vi "SQL_在指定表中指定字段插入多条数据.vi"(8 "error in (no error)":errorcluster caption="错误输入（无错误）", 9 "字段值(字符)":string[][](array[string]), 10 "字段名(字符)":string[](array[string]), 11 "表名":string="d7") -> (0 "error out":errorcluster caption="错误输出", 3 "SQL_在指定表中指定字段插入数据":string)   [LabVIEW 2014]
doc: "该模板用于创建子VI。"
uses:
  <vilib>/addons/database/NI_Database_API.lvlib
  <vilib>/addons/database/Connection.llb/DB Tools Open Connec (String).vi
  <vilib>/addons/database/Connection.llb/Conn Execute.vi
  <vilib>/addons/database/Recordset.llb/Rec Destroy - Connection.vi
panel:
  out "error out 2":errorcluster
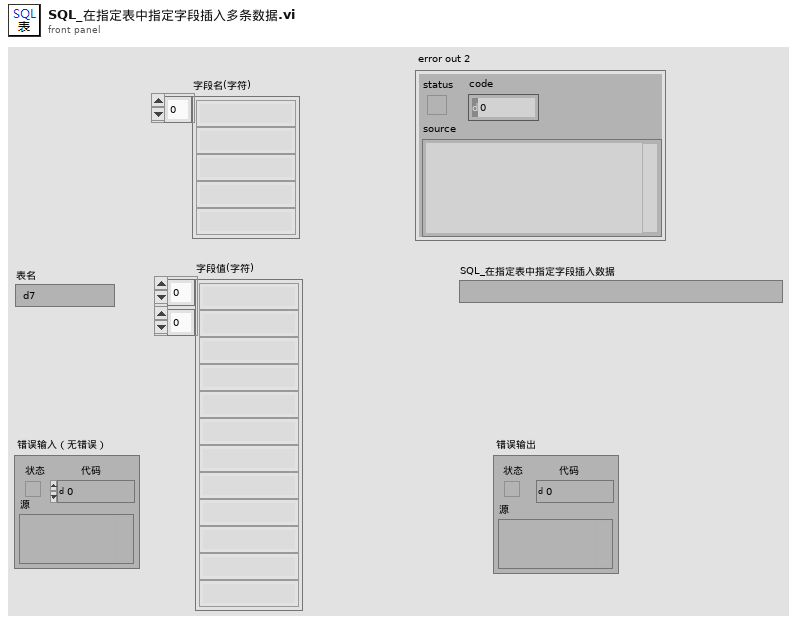
[diagram p1: front panel]
types:
  T1 = typedef "NI_Database_API.lvlib/Conn ObjectReference.ctl" = refnum<k1>
  T2 = typedef "NI_Database_API.lvlib/Rec ObjectReference.ctl" = refnum<k1>
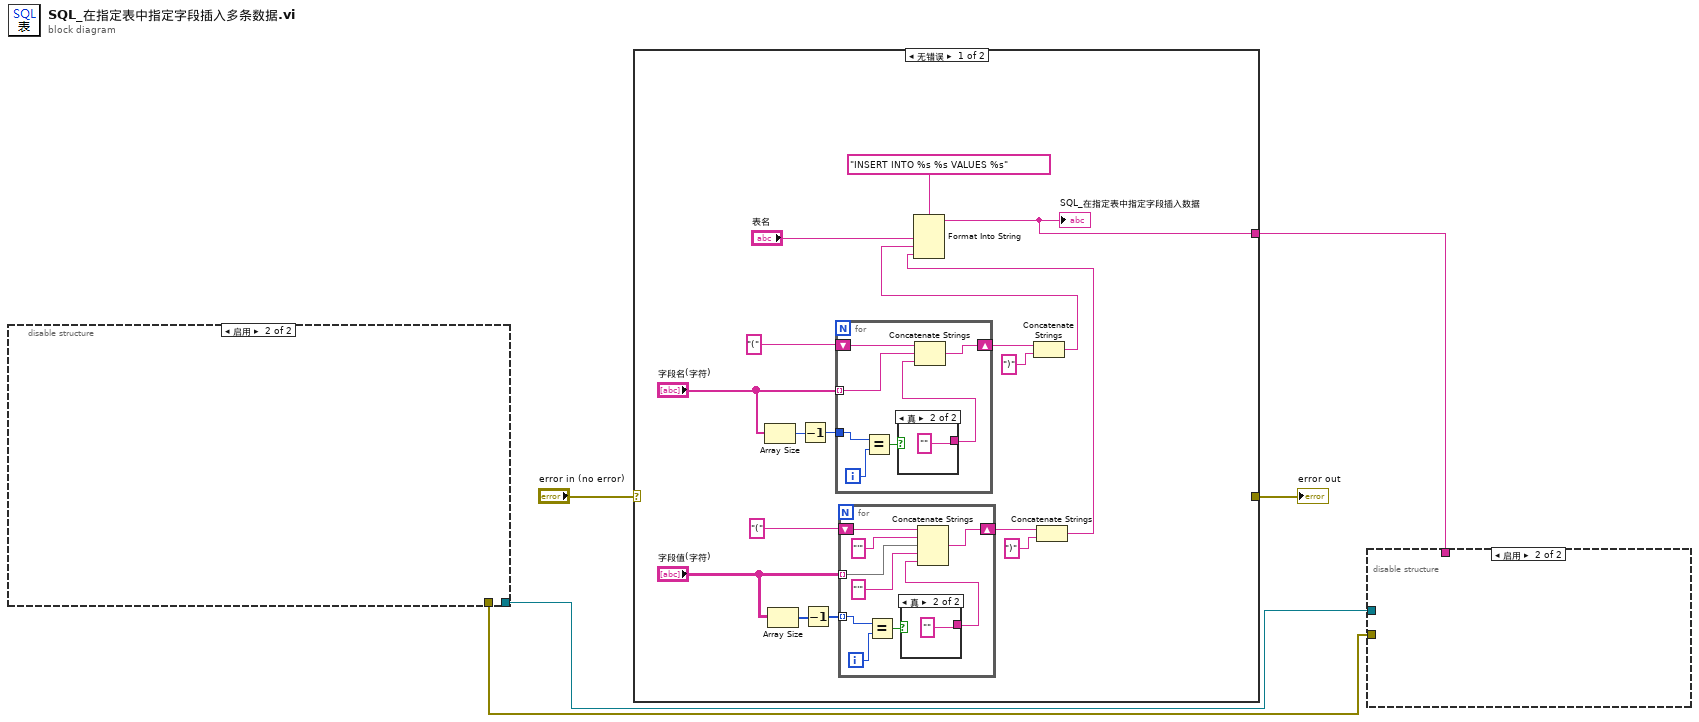
[diagram p0: block diagram]
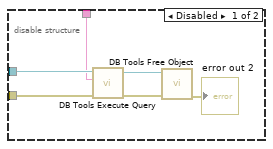
[diagram p2: hidden frame]
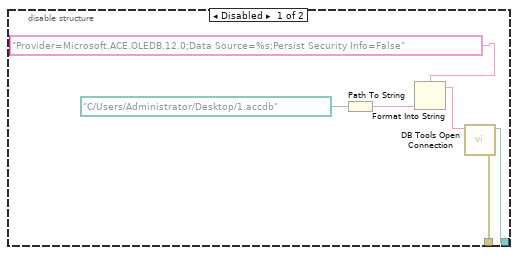
[diagram p3: hidden frame]
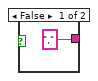
[diagram p4: hidden frame]
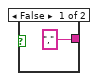
[diagram p5: hidden frame]
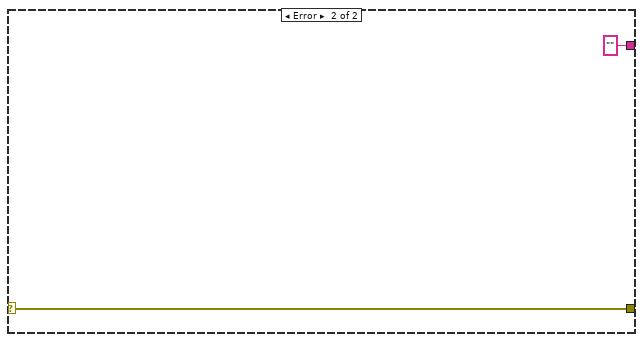
[diagram p6: hidden frame]
diagram:
  n1 = disable-structure shown="启用" {
    disable-tunnel: [w8 _] -> w3
    disable-tunnel: [w6 _] -> w2
    frame Disabled {
      n2 = Path To String(path=path "C:/Users/Administrator/Desktop/1.accdb" ("路径")) -> (string=w11:string)
      n3 = Format Into String(format string="Provider=Microsoft.ACE.OLEDB.12.0;Data Source=%s;Persist Security Info=False" ("初始字符串"), w11) -> (resulting string=w10:string)  [unwired: 2 in, 1 out]
      n4 = call-poly <vilib>:"DB Tools Open Connection.vi"("connection information"=w10) -> ("error out"=w6:errorcluster, "connection reference"=w8:T1)  [unwired: 7 in]
    }
    frame Enabled {
    }
  }
  n5 = case shown="无错误" "error in (no error)" {
    selector: "error in (no error)" -> [_ w50]
    tunnel: [_ w50] -> w4
    tunnel: [w12 ""] -> w1
    frame No Error {
      n6 = Array Size(array="字段名(字符)") -> (size(s)=w16:i32)
      n7 = Array Size(array="字段值(字符)") -> (size(s)=w24:i32[])
      n8 = Decrement(x=w16) -> (x-1=w17:i32)
      n9 = Decrement(x=w24) -> (x-1=w23:i32[])
      n10 = for {
        tunnel: "字段名(字符)" -> [w33] mode=indexing
        shift-right: [w34] -> w18
        shift-left: "(" -> [w35]
        tunnel: w17 -> [w30]
        i -> [w29]
        n11 = Equal?(x=w30, y=w29) -> (x = y?=w31:bool)
        n12 = case shown="真" w31 {
          tunnel: ["," ""] -> w32
          frame False {
          }
          frame True {
          }
        }
        n13 = Concatenate Strings(w35, w33, w32) -> (w34:string)
      }
      n14 = for {
        tunnel: "字段值(字符)" -> [w44] mode=indexing
        shift-right: [w45] -> w22
        shift-left: "(" -> [w46]
        tunnel: w23 -> [w39] mode=indexing
        i -> [w38]
        n15 = Equal?(x=w39, y=w38) -> (x = y?=w40:bool)
        n16 = case shown="真" w40 {
          tunnel: ["," ""] -> w41
          frame False {
          }
          frame True {
          }
        }
        n17 = Concatenate Strings(w46, "'", w44, "'", w41) -> (w45:string)
      }
      n18 = Concatenate Strings(w18, ")") -> (w13:string)
      n19 = Concatenate Strings(w22, ")") -> (w20:string)
      n20 = Format Into String(format string="INSERT INTO %s %s VALUES %s", "表名", w13, w20) -> (resulting string=w12:string)  [unwired: 2 in, 1 out]
      "SQL_在指定表中指定字段插入数据" <- w12
    }
    frame Error {
    }
  }
  "error out" <- w4
  n21 = disable-structure shown="启用" {
    disable-tunnel: w3 -> [w53 _]
    disable-tunnel: w2 -> [w52 _]
    disable-tunnel: w1 -> [w51 _]
    frame Disabled {
      n22 = call-poly <vilib>:"DB Tools Execute Query.vi"("error in (no error)"=w52, "SQL query"=w51, "connection reference"=w53) -> ("error out"=w55:errorcluster, "recordset reference"=w56:T2)  [unwired: 5 in]
      n23 = call-poly <vilib>:"DB Tools Free Object.vi"("error in (no error)"=w55, "recordset reference"=w56) -> ("error out"=→"error out 2":errorcluster)  [unwired: 8 in, 1 out]
    }
    frame Enabled {
    }
  }
